vi "sendScaledData.vi"(8 "error in (no error)":errorcluster, 11 "raw data":dbl) -> (0 "error out":errorcluster, 3 "weight":dbl)   [LabVIEW 2014]
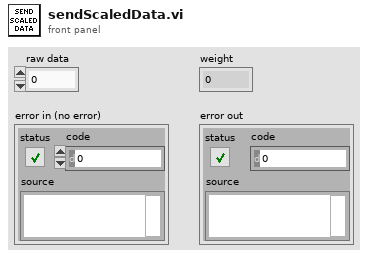
[diagram p1: front panel]
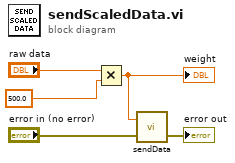
[diagram p0: block diagram]
diagram:
  n1 = Multiply(x="raw data", y=500.0) -> (x*y=w3:dbl)
  "weight" <- w3
  n2 = call "sendData.vi"("error in (no error)"="error in (no error)", "weight"=w3) -> ("error out"=→"error out":errorcluster)  [unwired: 1 in]
